vi "const dynamic file channel name.vi"() -> (3 "enable channel":string)   [LabVIEW 2018, in "TDMS datalogger configuration.lvclass"]
uses:
  TDMS datalogger configuration.lvclass
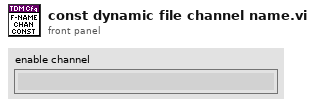
[diagram p1: front panel]
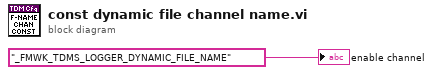
[diagram p0: block diagram]
diagram:
  "enable channel" <- "_FMWK_TDMS_LOGGER_DYNAMIC_FILE_NAME" ("enable channel")
